vi "Update Menu Controls Disable.vi"(8 "Error In":errorcluster, 9 "Enabled?":bool[](array[boolean]), 10 "Controls":refnum<vi>[](array[refnum]), 11 "State":enum16{"Init", "Update"}(ring)=enum."Update") -> (0 "Error Out":errorcluster)   [LabVIEW 2020, in "LMH-LINX.lvlib"]
uses:
  LMH-LINX.lvlib
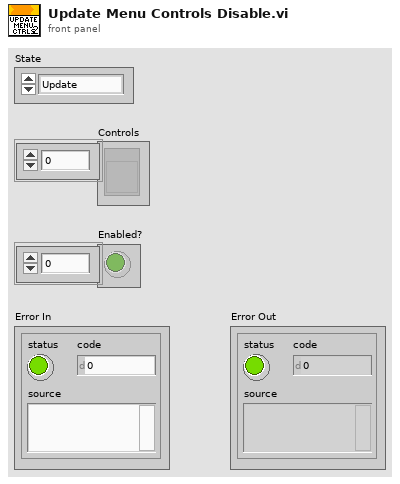
[diagram p1: front panel]
types:
  T1 = enum8{"Enabled", "Disabled", "Disabled and Grayed Out"}
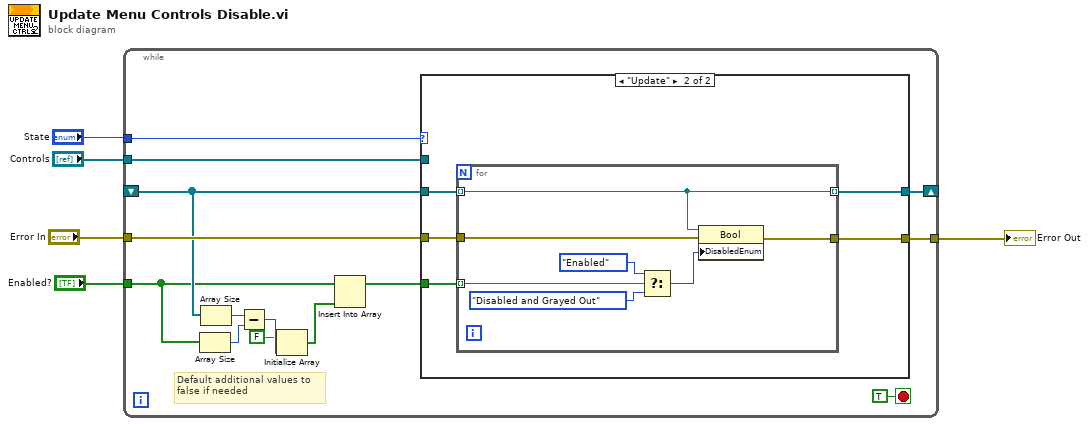
[diagram p0: block diagram]
diagram:
  n1 = while {
    shift-right: [w16] -> _
    shift-left: _ -> [w7]
    tunnel: "State" -> [w18]
    tunnel: "Controls" -> [w17]
    tunnel: [w15] -> w4
    tunnel: "Error In" -> [w14]
    tunnel: "Enabled?" -> [w6]
    stop <- TRUE stop-if-true
    # "Default additional values to \nfalse if needed"
    n2 = Array Size(array=w6) -> (size(s)=w11:i32)
    n3 = Array Size(array=w7) -> (size(s)=w10:i32)
    n4 = Subtract(x=w10, y=w11) -> (x-y=w12:i32)
    n5 = Initialize Array(FALSE, w12) -> (w13:bool[])
    n6 = Insert Into Array(array=w6, new element=w13) -> (w8:bool[])  [unwired: 1 in]
    n7 = case shown="\"Update\"" w18 {
      tunnel: [w21 w25] -> w16
      tunnel: w17 -> [w21 _]
      tunnel: w7 -> [_ w26]
      tunnel: [w20 w24] -> w15
      tunnel: w14 -> [w20 w23]
      tunnel: w8 -> [_ w22]
      frame "Init", Default {
      }
      frame "Update" {
        n8 = for {
          tunnel: w26 -> [w32] mode=indexing
          tunnel: [w33] -> w24
          tunnel: [w32] -> w25 mode=indexing
          tunnel: w23 -> [w31]
          tunnel: w22 -> [w30] mode=indexing
          n9 = Select(t=T1."Enabled" ("Disabled"), s=w30, f=T1."Disabled and Grayed Out" ("Disabled")) -> (s? t:f=w28:T1)
          n10 = property class="Bool"(reference=w32, error in=w31, "DisabledEnum"=w28) -> (error out=w33:errorcluster)  [unwired: 1 out]
        }
      }
    }
  }
  "Error Out" <- w4
